vi "GettingHistoricalData_Module.vi"() -> ()   [LabVIEW 2020]
uses:
  StateH.ctl
  V&T_Data.ctl
  D&P_Data.ctl
  <vilib>/Utility/file.llb/Read Delimited Spreadsheet (DBL).vi
panel:
  out "Sensor Locked?":bool
  out "Q OutOfRange?":bool
  out "Density and Pressure Graph":T1(graph)
  out "StateH":T2=enum."Wait"
  in  "Open Button":bool
  in  "stop":bool
  in  "Play Button":bool
  out "Viscosity and Temperature Graph":T1(graph)
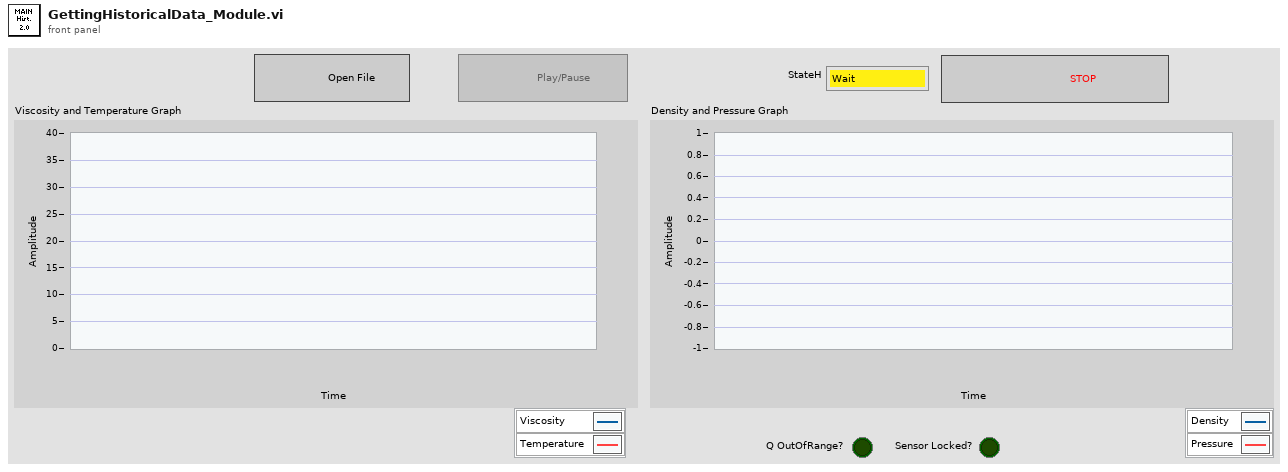
[diagram p1: front panel]
types:
  T1 = cluster{"seconds since 1Jan1904":timestamp, dbl, dbl}[]
  T2 = typedef "StateH.ctl" = enum16{"Initialize", "Wait", "OpenData", "Play", "Pause", "Finalize"}
  T3 = typedef "D&P_Data.ctl" = cluster{"time":timestamp, "Density":dbl, "Pressure":dbl}
  T4 = enum8{"Enabled", "Disabled", "Disabled and Grayed Out"}
  T5 = typedef "V&T_Data.ctl" = cluster{"time":timestamp, "Viscosity":dbl, "Temperature":dbl}
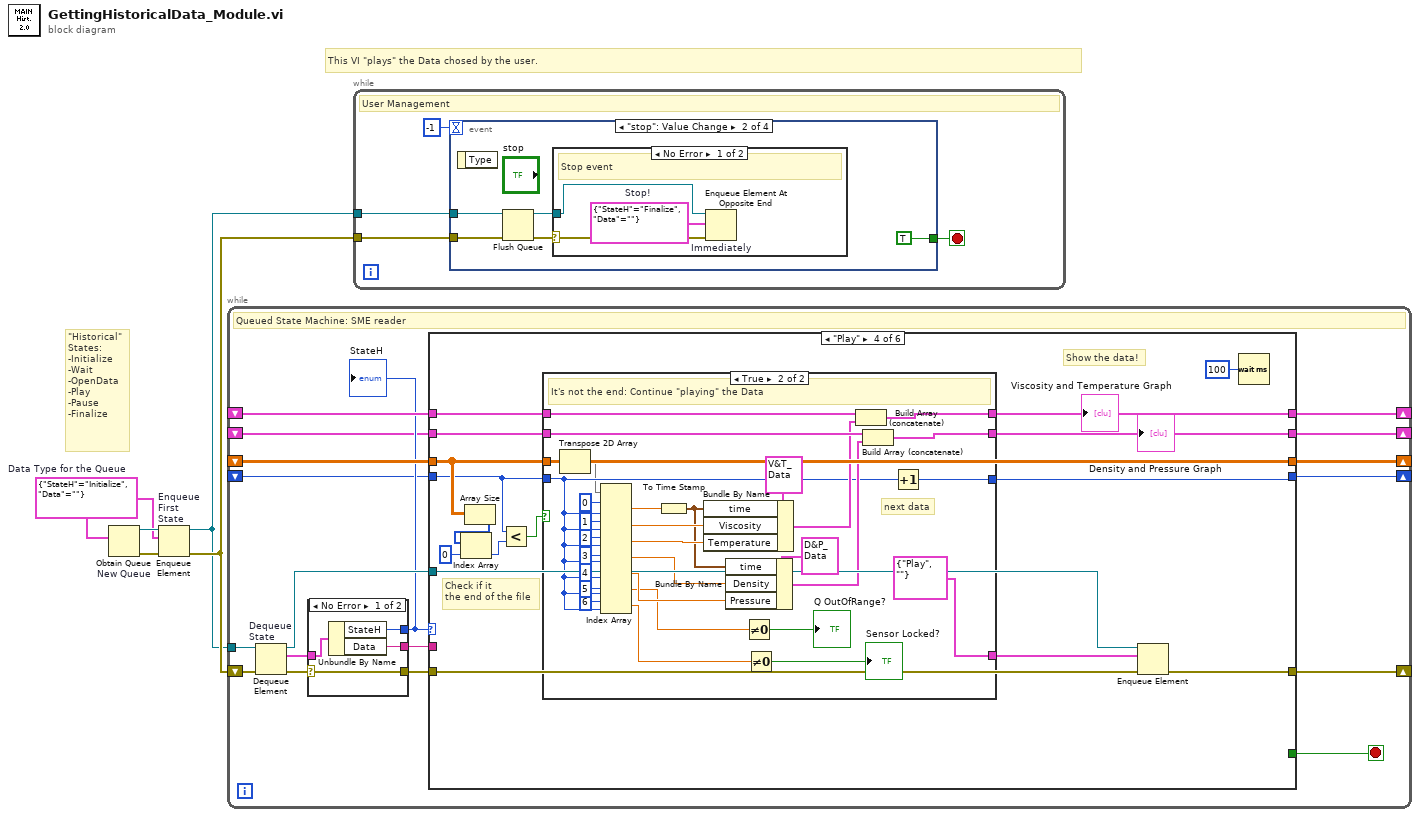
[diagram p0: block diagram]
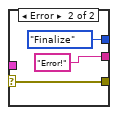
[diagram p2: hidden frame]
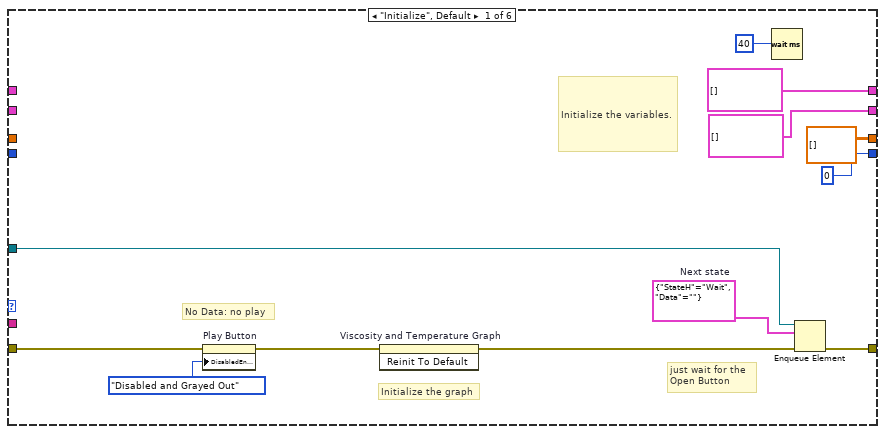
[diagram p3: hidden frame]
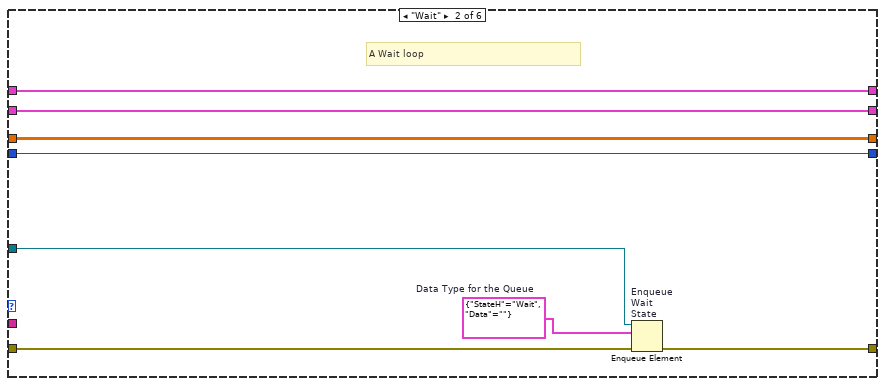
[diagram p4: hidden frame]
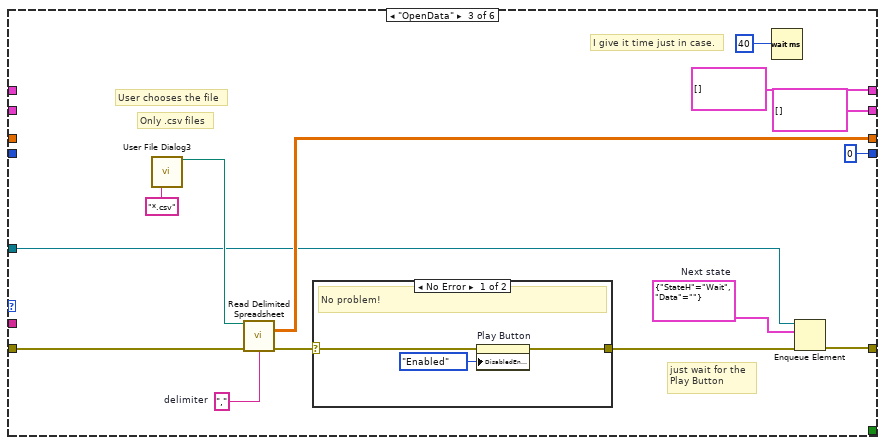
[diagram p5: hidden frame]
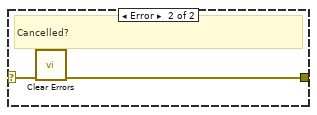
[diagram p6: hidden frame]
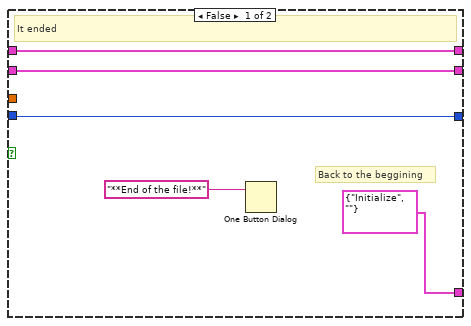
[diagram p7: hidden frame]
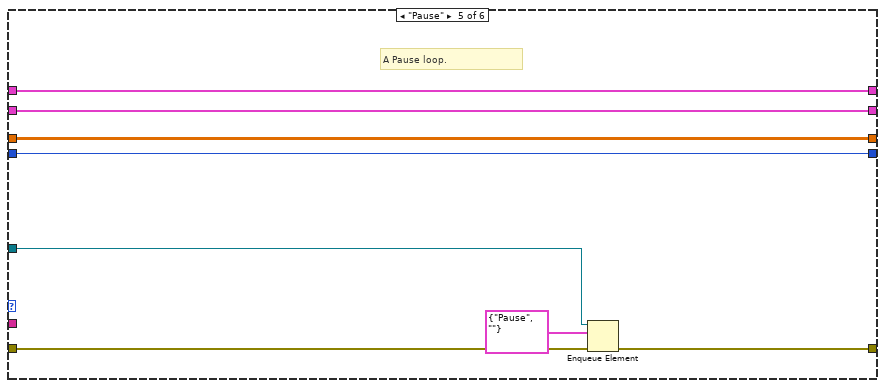
[diagram p8: hidden frame]
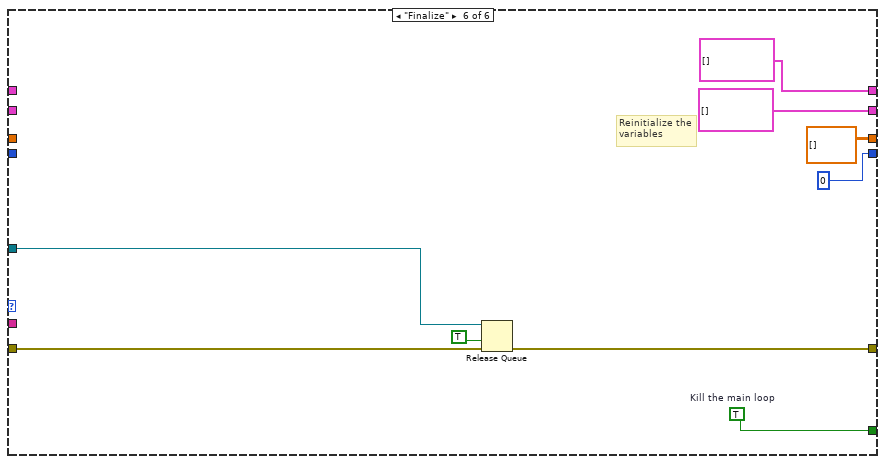
[diagram p9: hidden frame]
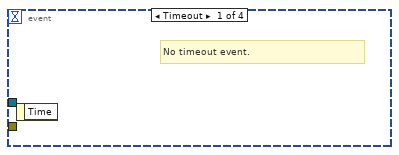
[diagram p10: hidden frame]
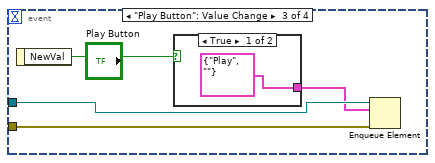
[diagram p12: hidden frame]
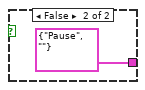
[diagram p13: hidden frame]
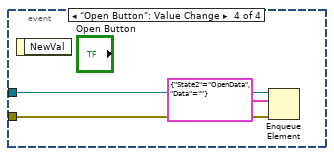
[diagram p14: hidden frame]
diagram:
  w4 = cluster{"StateH":T2, "Data":string} {"StateH"=enum."Initialize", "Data"=""}  # Data Type for the Queue
  # "This VI \"plays\" the Data chosed by the user."
  # "\"Historical\"\nStates:\n-Initialize\n-Wait\n-OpenData\n-Play\n-Pause\n-Finalize"
  n1 = Obtain Queue "New Queue"(element data type=w4) -> (queue out=w5:refnum<queue>, error out=w3:errorcluster)  [unwired: 4 in, 1 out]
  n2 = Enqueue Element "Enqueue\nFirst\nState"(queue=w5, element=w4, error in (no error)=w3) -> (queue out=w1:refnum<queue>, error out=w2:errorcluster)  [unwired: 1 in, 1 out]
  n3 = while {
    shift-right: [w21] -> _
    shift-left: w2 -> [w20]
    shift-right: [w14] -> _
    shift-left: _ -> [w15]
    shift-right: [w13] -> _
    shift-left: _ -> [w12]
    tunnel: w1 -> [w11]
    shift-right: [w8] -> _
    shift-left: _ -> [w9]
    shift-right: [w6] -> _
    shift-left: _ -> [w7]
    stop <- w17 stop-if-true
    # "Queued State Machine: SME reader"
    n4 = Dequeue Element "Dequeue\nState"(queue=w11, error in (no error)=w20) -> (queue out=w16:refnum<queue>, element=w18:cluster{"StateH":T2, "Data":string}, error out=w19:errorcluster)  [unwired: 1 in, 1 out]
    n5 = case shown="No Error" w19 {
      selector: w19 -> [w24 w29]
      tunnel: w18 -> [w27 _]
      tunnel: [w26 StateH."Finalize" ("StateH")] -> w10
      tunnel: [w25 "Error!" ("Data")] -> w23
      tunnel: [w24 w29] -> w22
      frame No Error {
        n6 = Unbundle By Name(w27) -> ("StateH"=w26:T2, "Data"=w25:string)
      }
      frame Error {
      }
    }
    "StateH" <- w10
    n7 = case shown="\"Play\"" w10 {
      tunnel: w23 -> [_ _ _ _ _ _]
      tunnel: w22 -> [w37 w46 w55 w82 w122 w133]
      tunnel: [w39 w45 w56 w80 w123 w136] -> w21
      tunnel: [_ _ _ _ _ w137] -> w17
      tunnel: w16 -> [w41 w48 w59 w81 w124 w135]
      tunnel: w15 -> [_ w50 _ w84 w126 _]
      tunnel: [T5[] [] w50 T5[] [] w83 w126 T5[] []] -> w14
      tunnel: [dbl[][] [] ("all rows") w49 w60 w78 w127 dbl[][] [] ("all rows")] -> w13
      tunnel: w12 -> [_ w49 _ w78 w127 _]
      tunnel: w9 -> [_ w44 _ w77 w128 _]
      tunnel: [0 w44 0 w79 w128 0] -> w8
      tunnel: w7 -> [_ w43 _ w71 w121 _]
      tunnel: [T3[] [] w43 T3[] [] w70 w121 T3[] []] -> w6
      frame "Initialize", Default {
        w40 = cluster{"StateH":T2, "Data":string} {"StateH"=enum."Wait", "Data"=""}  # Next state
        # "Initialize the graph"
        # "Initialize the variables."
        # "No Data: no play"
        # "just wait for the \nOpen Button"
        n8 = property on="Play Button" class="Bool"(error in=w37, "DisabledEnum"=T4."Disabled and Grayed Out" ("Disabled")) -> (error out=w34:errorcluster)  [unwired: 1 in, 1 out]
        n9 = invoke on="Viscosity and Temperature Graph" class="XYGraph (strict)" method="Reinit To Default"(error in=w34) -> (error out=w33:errorcluster)  [unwired: 2 in, 2 out]
        n10 = Wait (ms)(milliseconds to wait=u32 40) -> ()  [unwired: 1 out]
        n11 = Enqueue Element(queue=w41, element=w40, error in (no error)=w33) -> (error out=w39:errorcluster)  [unwired: 1 in, 2 out]
      }
      frame "Wait" {
        w47 = cluster{"StateH":T2, "Data":string} {"StateH"=enum."Wait", "Data"=""}  # Data Type for the Queue
        # "A Wait loop"
        n12 = Enqueue Element "Enqueue\nWait\nState"(queue=w48, element=w47, error in (no error)=w46) -> (error out=w45:errorcluster)  [unwired: 1 in, 2 out]
      }
      frame "OpenData" {
        w51 = ","  # delimiter
        w58 = cluster{"StateH":T2, "Data":string} {"StateH"=enum."Wait", "Data"=""}  # Next state
        # "I give it time just in case."
        # "Only .csv files"
        # "User chooses the file"
        # "just wait for the \nPlay Button"
        n13 = call "User File Dialog3"("pattern (all files)"="*.csv") -> ("selected path"=w61:path)  [unwired: 11 in, 3 out]
        n14 = call-poly <vilib>:"Read Delimited Spreadsheet.vi"("file path (dialog if empty)"=w61, "error in (no error)"=w55, "delimiter (\\t)"=w51) -> ("all rows"=w60:dbl[][], "error out"=w63:errorcluster)  [unwired: 7 in, 4 out]
        n15 = case shown="No Error" w63 {
          selector: w63 -> [w67 w69]
          tunnel: [w66 w68] -> w57
          frame No Error {
            # "No problem!"
            n16 = property on="Play Button" class="Bool"(error in=w67, "DisabledEnum"=T4."Enabled" ("Disabled")) -> (error out=w66:errorcluster)  [unwired: 1 in, 1 out]
          }
          frame Error {
            # "Cancelled?"
            n17 = call <vilib>:"Clear Errors.vi"("error in (no error)"=w69) -> ("error out"=w68:errorcluster)  [unwired: 5 in, 1 out]
          }
        }
        n18 = Wait (ms)(milliseconds to wait=u32 40) -> ()  [unwired: 1 out]
        n19 = Enqueue Element(queue=w59, element=w58, error in (no error)=w57) -> (error out=w56:errorcluster)  [unwired: 1 in, 2 out]
      }
      frame "Play" {
        # "Check if it\nthe end of the file"
        # "Show the data!"
        n20 = Array Size(array=w78) -> (size(s)=w76:i32[])
        n21 = Index Array(array=w76, index=0) -> (element=w74:i32)
        n22 = Less?(x=w77, y=w74) -> (x < y?=w73:bool)
        n23 = case shown="True" w73 {
          tunnel: w84 -> [w90 w120]
          tunnel: [w90 w116] -> w83
          tunnel: w78 -> [_ w115]
          tunnel: w77 -> [w89 w99]
          tunnel: [w89 w114] -> w79
          tunnel: [cluster{"State2":T2, "Data":string} {"State2"=enum."Initialize", "Data"=""} ("element") cluster{"State2":T2, "Data":string} {"State2"=enum."Play", "Data"=""} ("element")] -> w72
          tunnel: w71 -> [w86 w112]
          tunnel: [w86 w100] -> w70
          frame False {
            # "Back to the beggining"
            # "It ended"
            n24 = One Button Dialog(message="**End of the file!**") -> ()  [unwired: 1 in, 1 out]
          }
          frame True {
            # "next data"
            # "It's not the end: Continue \"playing\" the Data"
            n25 = Transpose 2D Array(2D array=w115) -> (transposed array=w91:dbl[][])
            n26 = Index Array(array=w91, index (row) #1=0 ("disabled index (row)"), index (col) #1=w99, index (row) #2=1 ("disabled index (row)"), index (col) #2=w99, index (row) #3=2 ("disabled index (row)"), index (col) #3=w99, index (row) #4=3 ("index (row)"), index (col) #4=w99, index (row) #5=4 ("index (row)"), index (col) #5=w99, index (row) #6=5 ("index (row)"), index (col) #6=w99, index (row) #7=6 ("disabled index (row)"), index (col) #7=w99) -> (element #1=w117:dbl, element #2=w107:dbl, element #3=w106:dbl, element #4=w103:dbl, element #5=w102:dbl, element #6=w97:dbl, element #7=w95:dbl)
            n27 = To Time Stamp(1:w117) -> (0:w93:timestamp)
            n28 = Bundle By Name(cluster=T5 {"time"=timestamp(0 s since 1904-01-01), "Viscosity"=0.0, "Temperature"=0.0} ("All Data"), "time"=w93, "Viscosity"=w107, "Temperature"=w106) -> (w105:T5)
            n29 = Bundle By Name(cluster=T3 {"time"=timestamp(0 s since 1904-01-01), "Density"=0.0, "Pressure"=0.0} ("D&P Data"), "time"=w93, "Density"=w103, "Pressure"=w102) -> (w101:T3)
            n30 = Not Equal To 0?(x=w97) -> (x != 0?=→"Q OutOfRange?":bool)
            n31 = Not Equal To 0?(x=w95) -> (x != 0?=→"Sensor Locked?":bool)
            n32 = Build Array (concatenate)(w120, w105) -> (w116:T5[])
            n33 = Build Array (concatenate)(w112, w101) -> (w100:T3[])
            n34 = Increment(x=w99) -> (x+1=w114:i32)
          }
        }
        "Viscosity and Temperature Graph" <- w83
        "Density and Pressure Graph" <- w70
        n35 = Enqueue Element(queue=w81, element=w72, error in (no error)=w82) -> (error out=w80:errorcluster)  [unwired: 1 in, 2 out]
        n36 = Wait (ms)(milliseconds to wait=u32 100) -> ()  [unwired: 1 out]
      }
      frame "Pause" {
        # "A Pause loop."
        n37 = Enqueue Element(queue=w124, element=cluster{"State2":T2, "Data":string} {"State2"=enum."Pause", "Data"=""}, error in (no error)=w122) -> (error out=w123:errorcluster)  [unwired: 1 in, 2 out]
      }
      frame "Finalize" {
        w137 = TRUE  # Kill the main loop
        # "Reinitialize the\nvariables"
        n38 = Release Queue(queue=w135, force destroy? (F)=TRUE, error in (no error)=w133) -> (error out=w136:errorcluster)  [unwired: 2 out]
      }
    }
  }
  n39 = while {
    tunnel: w2 -> [w139]
    tunnel: w1 -> [w138]
    stop <- w140 stop-if-true
    # "User Management"
    n40 = event shown="[1] \"stop\": Value Change" {
      selector: _ -> [_ _ _ _]
      dyn-events: _ -> [_ _ _ _]
      timeout: -1 -> [_ _ _ _]
      tunnel: [_ TRUE _ _] -> w140
      tunnel: w139 -> [_ w142 w150 w156]
      tunnel: w138 -> [_ w143 w152 w157]
      event Timeout {
        # "No timeout event."
        n41 = event-data() -> ()  [unwired: 1 in, 1 out]
      }
      event "stop": Value Change {
        n42 = event-data() -> ()  [unwired: 1 in, 1 out]
        n43 = Flush Queue(queue=w143, error in (no error)=w142) -> (queue out=w145:refnum<queue>, error out=w144:errorcluster)  [unwired: 1 out]
        n44 = case shown="No Error" w144 {
          selector: w144 -> [w148 _]
          tunnel: w145 -> [w149 _]
          frame No Error {
            w147 = cluster{"StateH":T2, "Data":string} {"StateH"=enum."Finalize", "Data"=""}  # Stop!
            # "Stop event"
            n45 = Enqueue Element At Opposite End "Immediately"(queue=w149, element=w147, error in (no error)=w148) -> ()  [unwired: 1 in, 3 out]
          }
          frame Error {
            # "Already dead"
          }
        }
      }
      event "Play Button": Value Change {
        n46 = event-data() -> ("NewVal"=w153:bool)  [unwired: 1 in]
        n47 = case shown="True" w153 {
          tunnel: [cluster{"State2":T2, "Data":string} {"State2"=enum."Play", "Data"=""} ("element") cluster{"State2":T2, "Data":string} {"State2"=enum."Pause", "Data"=""} ("element")] -> w151
          frame True {
          }
          frame False {
          }
        }
        n48 = Enqueue Element(queue=w152, element=w151, error in (no error)=w150) -> ()  [unwired: 1 in, 3 out]
      }
      event "Open Button": Value Change {
        n49 = event-data() -> ()  [unwired: 1 in, 1 out]
        n50 = Enqueue Element(queue=w157, element=cluster{"State2":T2, "Data":string} {"State2"=enum."OpenData", "Data"=""}, error in (no error)=w156) -> ()  [unwired: 1 in, 3 out]
      }
    }
  }
